vi "Motor_pwm_controle_de_posicao.vi"() -> ()   [LabVIEW 2018]
uses:
  <vilib>/Platform/TimedLoop/XDataNode/timing_clust.ctl
  <vilib>/Platform/TimedLoop/XDataNode/nitl_modes.ctl
  <vilib>/Platform/TimedLoop/XDataNode/wakeup.ctl
  <vilib>/platform/TimedLoop/XDataNode/XDataNode.xnode
  <vilib>/Platform/TimedLoop/XDataNode/XDNodeRunTimeDep.lvlib
panel:
  out "Diferença entre a posição atual e a desejada (°)":dbl
  out "Posição do motor":dbl[](graph)
  out "Aceleração":dbl[](graph)
  out "Velocidade de rotação do motor":dbl[](graph)
  in  "Taxa de convergência":dbl(slide) scale=0.0..5.0
  in  "Controle da posição":dbl(knob) scale=-60.0..60.0
  out "Sentido de Rotação":enum16{"Horário", "Anti-Horário"}(ring)
  in  "Tab Control":enum32{"Posição", "Velocidade", "Aceleração"}(tab)
  out "Posição Acumulada":waveform(dbl)(graph)
  out "Velocidade Acumulada":waveform(dbl)(graph)
  out "Aceleração acumulada":waveform(dbl)(graph)
  in  "Frequência do PWM (Hz)":dbl
  in  "stop":bool
  in  "Iniciar controle":bool
  in  "Tensão de alimentação (V)":dbl
  # "CONTROLE DE POSI敲O DE MOTOR DC"
  # "Controle de posição por PWM desenvolvido para um motor DC simulado"
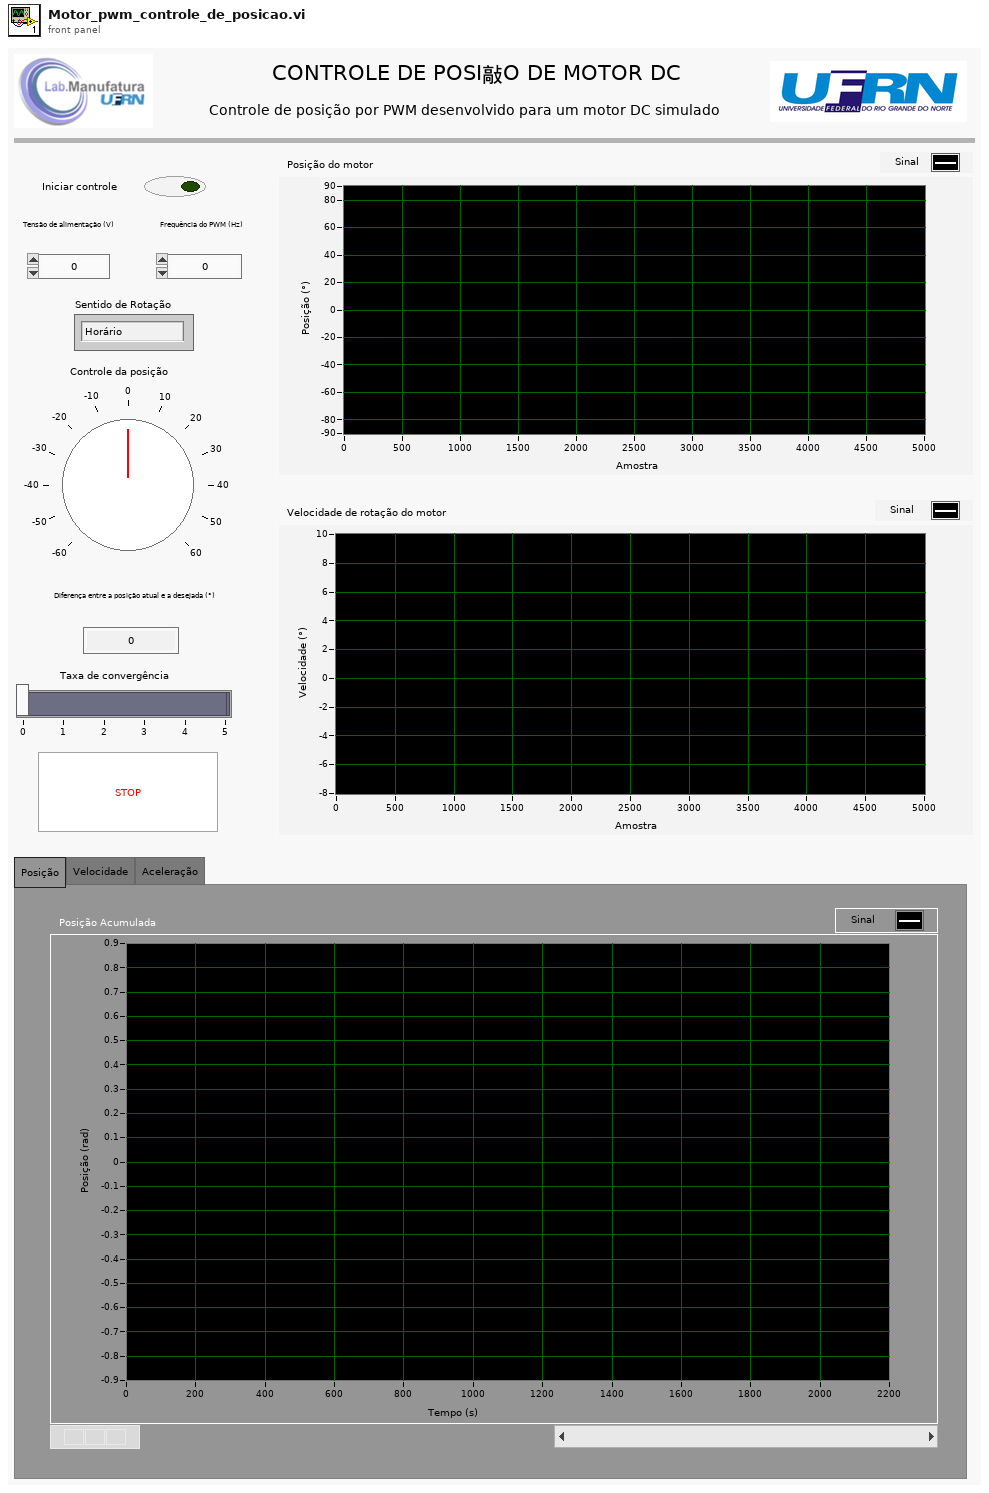
[diagram p1: front panel]
types:
  T1 = typedef "XDNodeRunTimeDep.lvlib/timing_clust.ctl" = cluster{"Expected End [f-1]":u64, "Actual End [f-1]":u64, "Finished Late? [f-1]":bool, "Expected End [i-1]":u64, "Actual End [i-1]":u64, "Finished Late? [i-1]":bool, "Expected Start [i]":u64, "Actual Start [i]":u64, "Expected Start [f]":u64, "Actual Start [f]":u64, "Source Name":string, "Structure Name":string, "Period":i64, "Deadline":i64, "Offset":i64, "Start":i64, "Priority":i32, "Timeout":i32, "Mode":T2, "Wakeup Reason":T3, "Error":errorcluster, "Source Type":string, "Secondary Source Type":string, "Global End Time":u64, "Global Start Time":u64, "Frame Duration":u64, "Iteration Duration":u64, "Assigned CPU":i32, "I/O Scan Engine Mode":u32}
  T2 = typedef "XDNodeRunTimeDep.lvlib/nitl_modes.ctl" = enum32{"No Change", "Process missed periods, maintain original phase", "Discard missed periods, maintain original phase", "Process missed periods, ignore original phase", "Discard missed periods, ignore original phase"}
  T3 = typedef "XDNodeRunTimeDep.lvlib/wakeup.ctl" = enum32{"Normal", "Aborted", "Asynchronous wakeup", "Timing source error", "Timed loop error", "Timeout"}
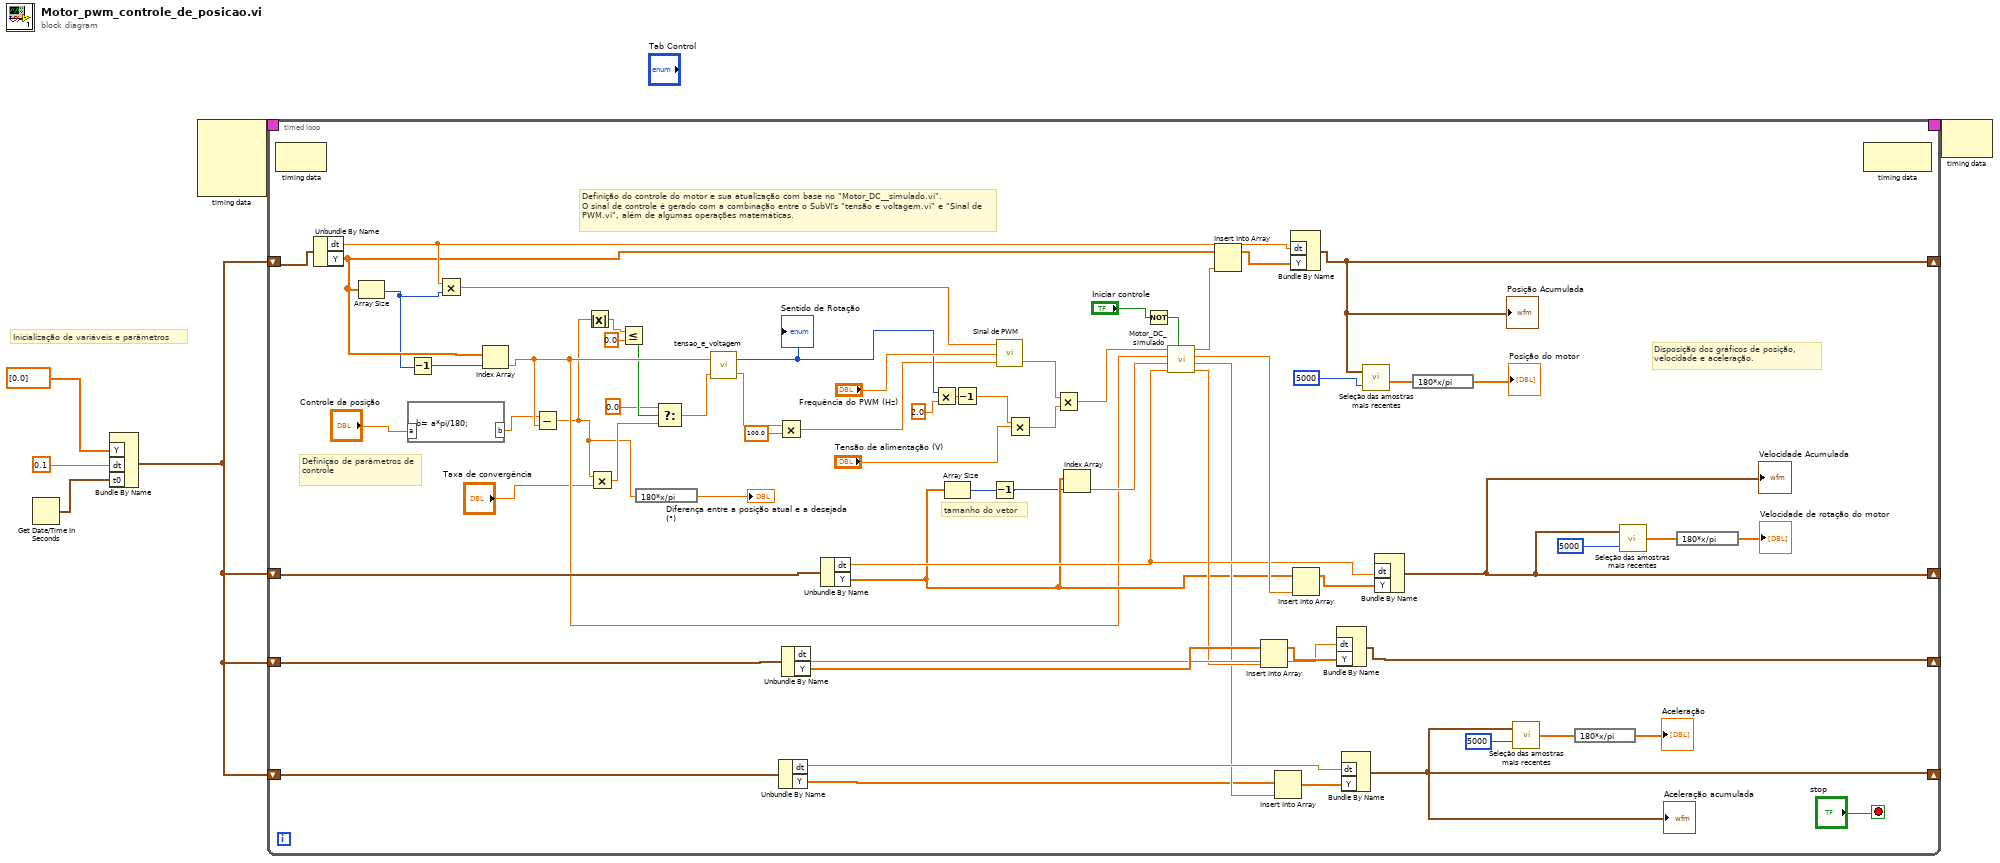
[diagram p0: block diagram]
diagram:
  # "Inicialização de variáveis e parâmetros"
  n1 = Get Date/Time In Seconds() -> (seconds since 1Jan1904=w3:timestamp)
  n2 = Bundle By Name("Y"=dbl[] [0.0], "dt"=0.1, "t0"=w3) -> (w1:waveform(dbl))  [unwired: 1 in]
  n3 = node-c288() -> (w6:T1)  [unwired: 4 in]
  n4 = timed-loop {
    shift-right: [w69] -> _
    shift-left: w1 -> [w70]
    shift-right: [w16] -> _
    shift-left: w1 -> [w72]
    shift-right: [w68] -> _
    shift-left: w1 -> [w71]
    shift-right: [w9] -> _
    shift-left: w1 -> [w67]
    timing: w6 -> [_]
    timing-out: [_] -> w5
    stop <- "stop" stop-if-true
    # "Disposição dos gráficos de posição, velocidade e aceleração."
    # "Definição do controle do motor e sua atualização com base no \"Motor_DC__simulado.vi\".\nO sinal de controle é gerado com a combinação entre o SubVI's \"tensão e voltagem.vi\" e \"Sinal de PWM.vi\", além de algumas operações matemáticas."
    # "Definiçao de parâmetros de controle"
    # "tamanho do vetor"
    n5 = node-c288() -> ()  [unwired: 1 in, 1 out]
    n6 = Unbundle By Name(w70) -> ("dt"=w37:dbl, "Y"=w35:dbl[])
    n7 = Array Size(array=w35) -> (size(s)=w17:i32)
    n8 = formula code="b= a*pi/180;"("a"="Controle da posição") -> ("b"=w30:dbl)
    n9 = Decrement(x=w17) -> (x-1=w36:i32)
    n10 = Multiply(x=w37, y=w17) -> (x*y=w33:dbl)
    n11 = Index Array(array=w35, index=w36) -> (element=w32:dbl)
    n12 = Subtract(x=w30, y=w32) -> (x-y=w7:dbl)
    n13 = Absolute Value(x=w7) -> (abs(x)=w25:dbl)
    n14 = Multiply(x=w7, y="Taxa de convergência") -> (x*y=w22:dbl)
    n15 = Less Or Equal?(x=w25, y=0.0) -> (x <= y?=w23:bool)
    n16 = expression code="180*x/pi"(w7) -> (→"Diferença entre a posição atual e a desejada (°)":dbl)
    n17 = Select(t=0.0, s=w23, f=w22) -> (s? t:f=w20:dbl)
    n18 = call "tensao_e_voltagem.vi"("T"=w20, "th"=w32) -> ("Duty Cycle"=w28:dbl, "Sentido"=w34:enum16{"Horário", "Anti-Horário"})
    "Sentido de Rotação" <- w34
    n19 = Multiply(x=w28, y=100.0) -> (x*y=w26:dbl)
    n20 = Unbundle By Name(w67) -> ("dt"=w44:dbl, "Y"=w41:dbl[])
    n21 = Unbundle By Name(w71) -> ("dt"=w61:dbl, "Y"=w63:dbl[])
    n22 = Unbundle By Name(w72) -> ("dt"=w47:dbl, "Y"=w40:dbl[])
    n23 = Multiply(x=w34, y=2.0) -> (x*y=w51:dbl)
    n24 = Array Size(array=w40) -> (size(s)=w39:i32)
    n25 = Decrement(x=w51) -> (x-1=w49:dbl)
    n26 = Decrement(x=w39) -> (x-1=w38:i32)
    n27 = call "Sinal de PWM.vi"("duty cycle"=w26, "Frequência do PWM"="Frequência do PWM (Hz)", "Tempo atual"=w33) -> ("Resultado numérico"=w56:dbl)  [unwired: 1 out]
    n28 = Multiply(x=w49, y="Tensão de alimentação (V)") -> (x*y=w48:dbl)
    n29 = Multiply(x=w56, y=w48) -> (x*y=w55:dbl)
    n30 = Index Array(array=w40, index=w38) -> (element=w46:dbl)
    n31 = Not(x="Iniciar controle") -> (.not. x?=w19:bool)
    n32 = call "Motor_DC_simulado.vi"("Initialize"=w19, "dt"=w47, "Velocidade anterior"=w46, "Posiçao anterior"=w32, "DC_Vin"=w55) -> ("Tensão fornecida ao motor"=w60:dbl, "Aceleração"=w43:dbl, "Velocidade"=w59:dbl, "Posição"=w58:dbl)  [unwired: 2 in]
    n33 = Insert Into Array(array=w35, new element=w58) -> (w65:dbl[])  [unwired: 1 in]
    n34 = Insert Into Array(array=w63, new element=w60) -> (w62:dbl[])  [unwired: 1 in]
    n35 = Insert Into Array(array=w41, new element=w43) -> (w45:dbl[])  [unwired: 1 in]
    n36 = Bundle By Name("dt"=w37, "Y"=w65) -> (w69:waveform(dbl))  [unwired: 1 in]
    "Posição Acumulada" <- w69
    n37 = Insert Into Array(array=w40, new element=w59) -> (w64:dbl[])  [unwired: 1 in]
    n38 = Bundle By Name("dt"=w61, "Y"=w62) -> (w68:waveform(dbl))  [unwired: 1 in]
    n39 = Bundle By Name("dt"=w44, "Y"=w45) -> (w9:waveform(dbl))  [unwired: 1 in]
    "Aceleração acumulada" <- w9
    n40 = call "Seleção das amostras mais recentes.vi"("Número de amostras no gráfico"=5000, "Vetor de entrada"=w69) -> ("Amostras do gráfico"=w14:dbl[])
    n41 = Bundle By Name("dt"=w47, "Y"=w64) -> (w16:waveform(dbl))  [unwired: 1 in]
    "Velocidade Acumulada" <- w16
    n42 = expression code="180*x/pi"(w14) -> (→"Posição do motor":dbl[])
    n43 = call "Seleção das amostras mais recentes.vi"("Número de amostras no gráfico"=5000 ("Número de amostras no gráfico 2"), "Vetor de entrada"=w9) -> ("Amostras do gráfico"=w11:dbl[])
    n44 = expression code="180*x/pi"(w11) -> (→"Aceleração":dbl[])
    n45 = call "Seleção das amostras mais recentes.vi"("Número de amostras no gráfico"=5000 ("Número de amostras no gráfico 2"), "Vetor de entrada"=w16) -> ("Amostras do gráfico"=w13:dbl[])
    n46 = expression code="180*x/pi"(w13) -> (→"Velocidade de rotação do motor":dbl[])
    n47 = node-c288() -> ()  [unwired: 1 in, 1 out]
  }
  n48 = node-c288(w5) -> ()  [unwired: 1 out]
